vi "Get TableName.vi"(8 "error in (no error)":errorcluster, 11 "NI_DB_API in":refnum<class "NI_DB_API.lvclass">) -> (0 "error out":errorcluster, 2 "TableName List":string[](array[string]), 3 "NI_DB_API out":refnum<class "NI_DB_API.lvclass">)   [LabVIEW 2021, in "NI_DB_API.lvclass"]
uses:
  <userlib>/John_Lib/DataBase/NI_DB_API/NI_DB_API.lvclass
  <userlib>/John_Lib/DataBase/NI_DB_API/NI_DB_API.lvclass/NI_DB_API.ctl
  <vilib>/addons/database/NI_Database_API.lvlib
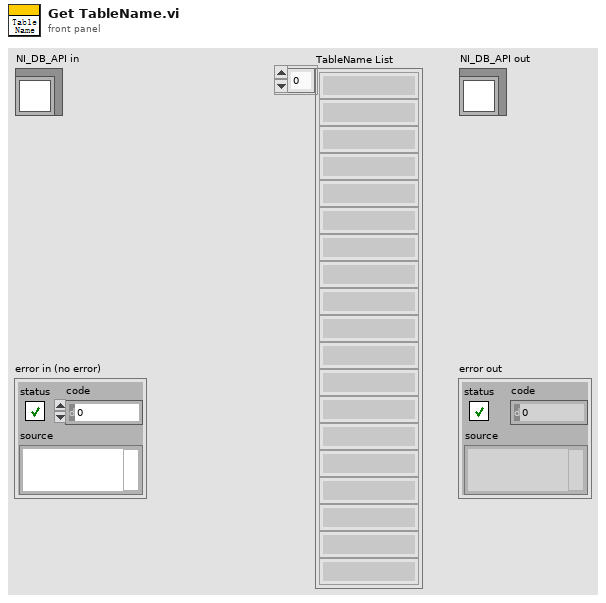
[diagram p1: front panel]
types:
  T1 = typedef "NI_Database_API.lvlib/Conn ObjectReference.ctl" = refnum<k1>
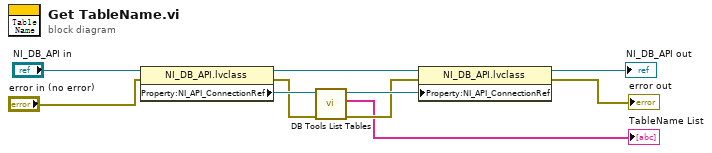
[diagram p0: block diagram]
diagram:
  n1 = property class="NI_DB_API.lvclass"(reference="NI_DB_API in", error in="error in (no error)") -> (reference out=w10:refnum<class "NI_DB_API.lvclass">, error out=w3:errorcluster, "Property:NI_API_ConnectionRef"=w5:T1)
  n2 = call <vilib>:"DB Tools List Tables.vi"("error in (no error)"=w3, "connection reference"=w5) -> ("error out"=w2:errorcluster, "tables"=→"TableName List":string[], "connection reference out"=w4:T1)  [unwired: 3 in]
  n3 = property class="NI_DB_API.lvclass"(reference=w10, error in=w2, "Property:NI_API_ConnectionRef"=w4) -> (reference out=→"NI_DB_API out":refnum<class "NI_DB_API.lvclass">, error out=→"error out":errorcluster)
